vi "CopyArrayToImageARGBPixels.vi"(8 "error in (no error)":errorcluster, 10 "ARGB Image Destination":refnum<data-value>, 11 "Source":u8[][][](array[numeric])) -> (0 "error out":errorcluster, 3 "ARGB Image Destination (Duplicate)":refnum<data-value>)   [LabVIEW 2020, in "g_ar_toolkit.image.lvlib"]
uses:
  g_ar_toolkit.image.lvlib
  g_ar_toolkit.common/Image Size (Integer).ctl
  g_ar_toolkit.common/g_ar_toolkit.common.lvlib
  bin/g_ar_toolkit.1.32.dll
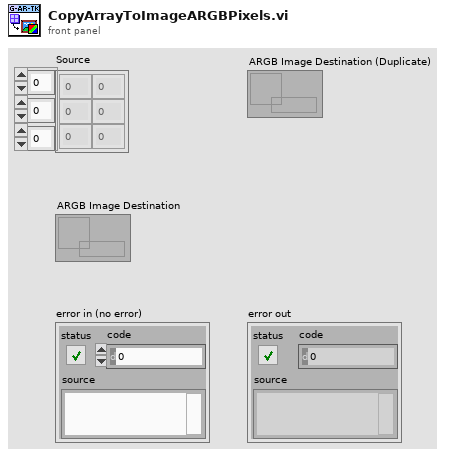
[diagram p1: front panel]
types:
  T1 = typedef "g_ar_toolkit.common.lvlib/Image Size (Integer).ctl" = cluster{"Width":u16, "Height":u16}
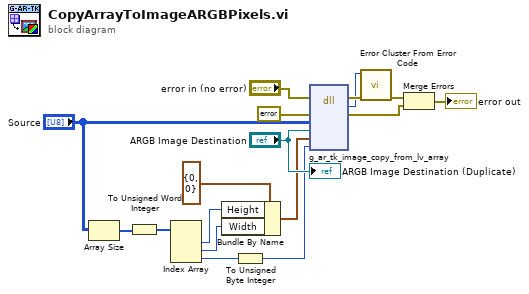
[diagram p0: block diagram]
diagram:
  n1 = Array Size(array="Source") -> (size(s)=w9:i32[])
  n2 = To Unsigned Word Integer(number=w9) -> (unsigned 16bit integer=w8:u16[])
  n3 = Index Array(array=w8) -> (element #1=w4:u16, element #2=w3:u16, element #3=w7:u16)  [unwired: 3 in]
  n4 = Bundle By Name(cluster=T1 {"Width"=0, "Height"=0} ("Image Size"), "Height"=w4, "Width"=w3) -> (w2:T1)
  n5 = To Unsigned Byte Integer(number=w7) -> (unsigned 8bit integer=w6:u8)
  n6 = dll-call lib="C:/serenial/libraries/g-augmented-reality-toolkit/LabVIEW/bin/g_ar_toolkit.1.*.*" fn="g_ar_tk_image_copy_from_lv_array" ("g_ar_toolkit.*.*:g_ar_tk_image_copy_from_raw_memory")(error in="error in (no error)", "error_cluster"=errorcluster {"status"=FALSE, "code"=0, "source"=""} ("error constant"), "Source"="Source", "EDVR Dst"="ARGB Image Destination", "Size"=w2, "array third dim"=w6) -> (error out=w11:errorcluster, "MgErr"=w10:i32, "error_cluster"=w16:errorcluster)  [unwired: 6 in, 1 out]
  n7 = call <vilib>:"Error Cluster From Error Code.vi"("error in (no error)"=w11, "error code (0)"=w10) -> ("error out"=w12:errorcluster)  [unwired: 7 in]
  n8 = Merge Errors(w12, w16) -> (→"error out":errorcluster)
  "ARGB Image Destination (Duplicate)" <- "ARGB Image Destination"
